vi "WS1021 CP Voltages Setting.vi"(6 "Select CPV":i32(ring) items=["CP OFF", "CP ON", "OTP OFF", "CP 24V", "CP 26V", "CP 28V", "CP 30V", "CP 31V", "CP 32V", "CP 33V", "CP 34V", "CP 35V", "CP 36V", "CP 37V", "CP 38V", "CP 39V", "CP 40V", "CP 41V", "CP 42V", "CP 43V", "CP 44V", "CP 45V", "CP 46V", "CP 47V", "CP 48V", "CP 49V", "CP 50V", "CP 51V", "CP 52V", "CP 53V", "CP 54V", "CP 56V", "CP 58V", "CP 60V", "CP 62V"], 7 "CP For Test":dbl[](array[numeric]), 8 "Error In":errorcluster) -> (0 "Error Out":errorcluster, 1 "Cmd Select":string[](array[string]), 2 "CP Select":string, 3 "Cmd Send out":string, 4 "Multi CP Select":i32[](array[numeric]), 5 "List CP":string[](array[string]))   [LabVIEW 2017]
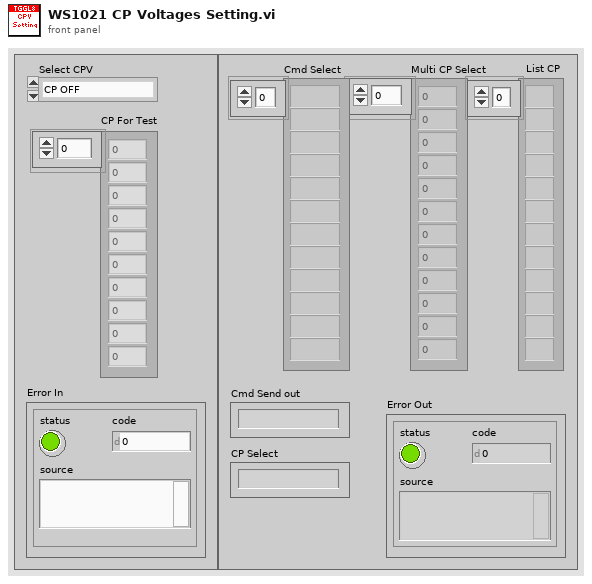
[diagram p1: front panel]
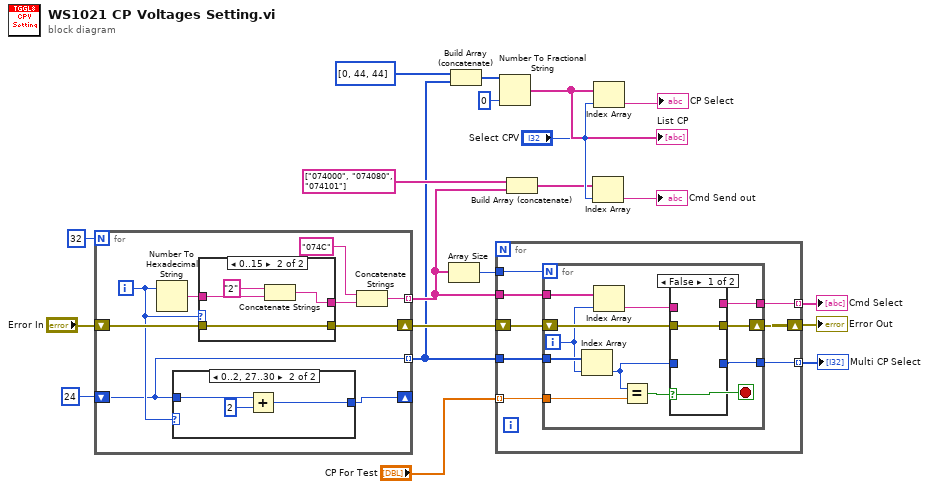
[diagram p0: block diagram]
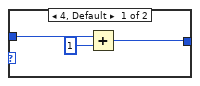
[diagram p3: hidden frame]
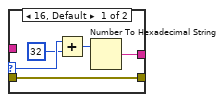
[diagram p4: hidden frame]
diagram:
  n1 = for {
    N: 32 -> [_]
    tunnel: [w28] -> w5 mode=indexing
    shift-right: [w24] -> w17
    shift-left: "Error In" -> [w25]
    shift-right: [w21] -> _
    shift-left: 24 -> [w22]
    tunnel: [w22] -> w1 mode=indexing
    i -> [w23]
    n2 = Number To Hexadecimal String(2:w23) -> (0:w29:string)  [unwired: 1 in]
    n3 = case shown="0..2, 27..30" w23 {
      tunnel: w22 -> [w32 w35]
      tunnel: [w30 w33] -> w21
      frame 4, Default {
        n4 = Add(x=w32, y=1) -> (x+y=w30:i32)
      }
      frame 0..2, 27..30 {
        n5 = Add(x=w35, y=2) -> (x+y=w33:i32)
      }
    }
    n6 = case shown="0..15" w23 {
      selector: w23 -> [w40 _]
      tunnel: w29 -> [_ w43]
      tunnel: [w38 w42] -> w27
      tunnel: w25 -> [w36 w41]
      tunnel: [w36 w41] -> w24
      frame 16, Default {
        n7 = Add(x=w40, y=32) -> (x+y=w39:i32)
        n8 = Number To Hexadecimal String(2:w39) -> (0:w38:string)  [unwired: 1 in]
      }
      frame 0..15 {
        n9 = Concatenate Strings("2" ("string"), w43) -> (w42:string)
      }
    }
    n10 = Concatenate Strings("074C" ("string"), w27) -> (w28:string)
  }
  n11 = Array Size(array=w5) -> (size(s)=w12:i32)
  n12 = Build Array (concatenate)(i32[] [0, 44, 44], w1) -> (w2:i32[])
  n13 = for {
    shift-right: [w50] -> w16
    shift-left: w17 -> [w51]
    tunnel: w5 -> [w48]
    tunnel: w1 -> [w49]
    tunnel: "CP For Test" -> [w52] mode=indexing
    tunnel: [w46] -> w14 mode=indexing
    tunnel: [w47] -> w13 mode=indexing
    tunnel: w12 -> [w45]
    n14 = for {
      N: w45 -> [_]
      tunnel: w52 -> [w63]
      shift-right: [w61] -> w50
      shift-left: w51 -> [w62]
      tunnel: w49 -> [w60]
      tunnel: w48 -> [w57]
      tunnel: [w55] -> w47
      tunnel: [w54] -> w46
      i -> [w58]
      stop <- w53 stop-if-true
      n15 = Index Array(array=w60, index=w58) -> (element=w59:i32)
      n16 = Index Array(array=w57, index=w58) -> (element=w56:string)
      n17 = Equal?(x=w59, y=w63) -> (x = y?=w53:bool)
      n18 = case shown="False" w53 {
        tunnel: w62 -> [w64 w66]
        tunnel: w56 -> [_ w67]
        tunnel: [_ w67] -> w55
        tunnel: w59 -> [_ w65]
        tunnel: [_ w65] -> w54
        tunnel: [w64 w66] -> w61
        frame False {
        }
        frame True {
        }
      }
    }
  }
  "Error Out" <- w16
  "Multi CP Select" <- w14
  "Cmd Select" <- w13
  n19 = Number To Fractional String(number=w2, precision (6)=i16 0) -> (F-format string=w9:string[])  [unwired: 2 in]
  "List CP" <- w9
  n20 = Build Array (concatenate)(string[] ["074000", "074080", "074101"], w5) -> (w4:string[])
  n21 = Index Array(array=w4, index="Select CPV") -> (element=→"Cmd Send out":string)
  n22 = Index Array(array=w9, index="Select CPV") -> (element=→"CP Select":string)
